vi "UTILITY DBL Array to String Array.vi"(8 "Error in (no error)":errorcluster, 11 "Array in":dbl[][](array[numeric])) -> (0 "Error out":errorcluster, 3 "String array out":string="[1,23-2-3]\n[4-3,22-2]\n[3-4,01-8]\n[0-7-6,66]")   [LabVIEW 2014]
panel:
  # "Double array to string array"
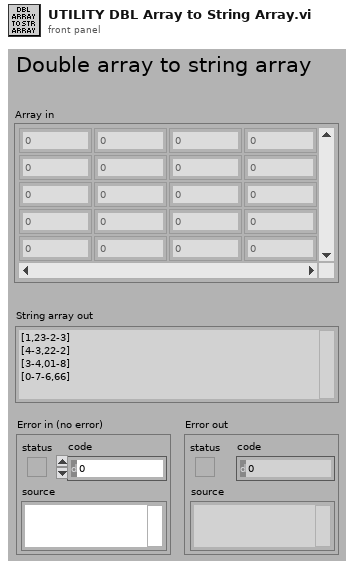
[diagram p1: front panel]
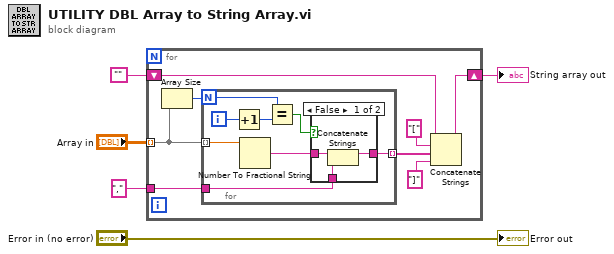
[diagram p0: block diagram]
diagram:
  n1 = for {
    tunnel: "Array in" -> [w12] mode=indexing
    shift-right: [w11] -> w2
    shift-left: "" -> [w10]
    tunnel: "," ("Delimiter") -> [w6]
    n2 = Array Size(array=w12) -> (size(s)=w13:i32)
    n3 = for {
      N: w13 -> [w20]
      tunnel: w12 -> [w17] mode=indexing
      tunnel: [w15] -> w7 mode=indexing
      tunnel: w6 -> [w14]
      i -> [w21]
      n4 = Increment(x=w21) -> (x+1=w19:i32)
      n5 = Number To Fractional String(number=w17) -> (F-format string=w16:string)  [unwired: 3 in]
      n6 = Equal?(x=w20, y=w19) -> (x = y?=w18:bool)
      n7 = case shown="False" w18 {
        tunnel: w16 -> [w23 w25]
        tunnel: [w24 w25] -> w15
        tunnel: w14 -> [w22 _]
        frame False {
          n8 = Concatenate Strings(w23, w22) -> (w24:string)
        }
        frame True {
        }
      }
    }
    n9 = Concatenate Strings(w10, "[" ("string"), w7, "]" ("string")) -> (w11:string)
  }
  "String array out" <- w2
  "Error out" <- "Error in (no error)"
